vi "RW XY graph.vi"(0 "reference in":refnum<class "XYgraph.lvclass">, 1 "XY in":cluster{"X":dbl[], "Y":dbl[]}[](array[cluster]), 3 "Write (F)":bool, 5 "error in (no error)":errorcluster) -> (14 "reference out":refnum<class "XYgraph.lvclass">, 15 "XY out":cluster{"X":dbl[], "Y":dbl[]}[](array[cluster]), 19 "error out":errorcluster)   [LabVIEW 2019, in "XYgraph.lvclass"]
doc: "Reads and writes data to the xy graph reference"
uses:
  XYgraph.lvclass
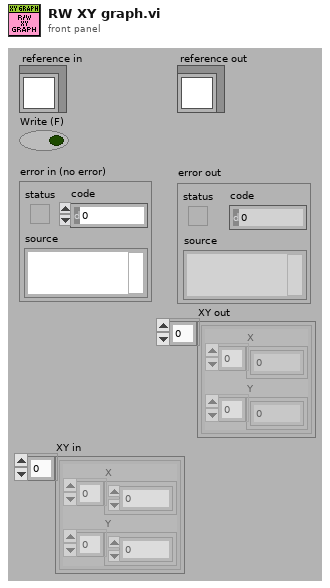
[diagram p1: front panel]
types:
  T1 = typedef "XYgraph.lvclass/ObjectAttributes.ctl" = cluster{"FPref":T2, "MyAttribute":dbl, "X multiplier":dbl, "Y multiplier":dbl, "X Scale name":string, "Y Scale name":string, "Fcurve metadata":T3, "Fcurve":refnum<class "Fcurve.lvclass">}
  T2 = typedef "XYgraph.lvclass/XY graph ref.ctl" = refnum<vi>
  T3 = typedef "Fcurve.lvclass/Metadata.ctl" = cluster{"dt (us)":dbl, "Dec Factor":dbl, "Z piezo Sensitivity (nm/V)":dbl, "K (N/m)":dbl, "Sp (V)":dbl, "Contact (ms)":dbl, "Zpos contact":dbl, "Vel_app (nm/s)":dbl, "Vel_ret (nm/s)":dbl, "deltaV (nm)":dbl, "Def_V0 (v)":dbl, "Piezo gain":dbl, "invOLS (nm/V)":dbl}
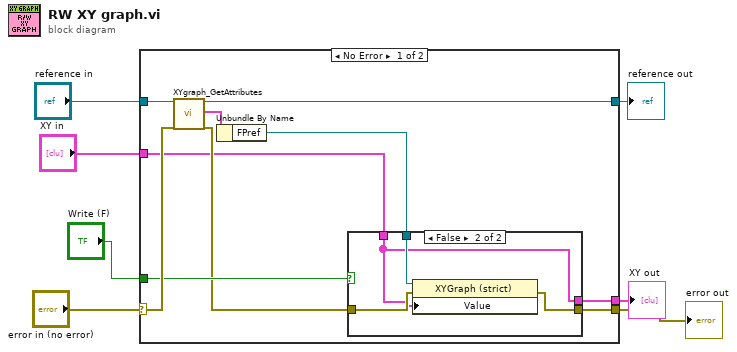
[diagram p0: block diagram]
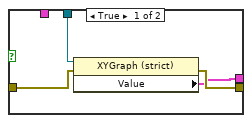
[diagram p2: hidden frame]
diagram:
  n1 = case shown="No Error" "error in (no error)" {
    selector: "error in (no error)" -> [w17 w28]
    tunnel: [w15 w28] -> w6
    tunnel: [w10 w27] -> w4
    tunnel: "reference in" -> [w16 w27]
    tunnel: "Write (F)" -> [w14 _]
    tunnel: [w12 w26] -> w2
    tunnel: "XY in" -> [w11 w26]
    frame No Error {
      n2 = call "XYgraph_GetAttributes.vi"("reference in"=w16, "error in (no error)"=w17) -> ("reference out"=w10:refnum<class "XYgraph.lvclass">, "attributes"=w9:T1, "error out"=w13:errorcluster)  [unwired: 14 in, 1 out]
      n3 = Unbundle By Name(w9) -> ("FPref"=w8:T2)
      n4 = case shown="False" w14 {
        tunnel: w8 -> [w21 w25]
        tunnel: w13 -> [w20 w24]
        tunnel: [w19 w23] -> w15
        tunnel: [w18 w22] -> w12
        tunnel: w11 -> [_ w22]
        frame True {
          n5 = property class="XYGraph (strict)"(reference=w21, error in=w20) -> (error out=w19:errorcluster, "Value"=w18:cluster{"X":dbl[], "Y":dbl[]}[])  [unwired: 1 out]
        }
        frame False {
          n6 = property class="XYGraph (strict)"(reference=w25, error in=w24, "Value"=w22) -> (error out=w23:errorcluster)  [unwired: 1 out]
        }
      }
    }
    frame Error {
    }
  }
  "error out" <- w6
  "reference out" <- w4
  "XY out" <- w2
